vi "Open PolarizationProcessor.vi"(8 "error in (no error)":errorcluster, 11 "PolarizationProcessorSDK reference":refnum<k24>) -> (0 "error out":errorcluster, 2 "PolarizationProcessor reference":refnum<k24>, 3 "PolarizationProcessorSDK reference out":refnum<k24>)   [LabVIEW 2015]
uses:
  C:/code/Host/Installer/Scientific Camera Interfaces/LabVIEW/32_bit/Library_X86/Thorlabs.TSI.PolarizationProcessor.dll
  code/Host/Installer/Scientific Camera Interfaces/LabVIEW/32_bit/Library_X86/Thorlabs.TSI.PolarizationProcessor.dll
  C:/code/Host/Installer/Scientific Camera Interfaces/LabVIEW/32_bit/Library_X86/Thorlabs.TSI.PolarizationInterfaces.dll
  code/Host/Installer/Scientific Camera Interfaces/LabVIEW/32_bit/Library_X86/Thorlabs.TSI.PolarizationInterfaces.dll
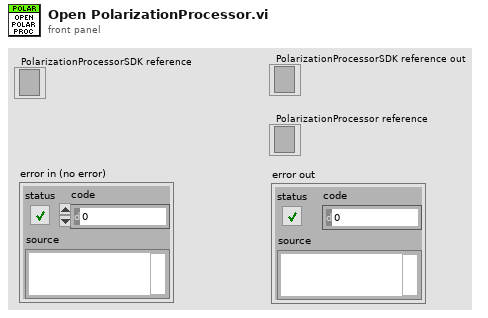
[diagram p1: front panel]
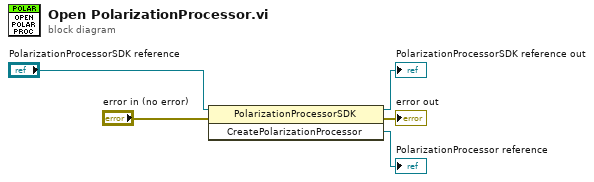
[diagram p0: block diagram]
diagram:
  n1 = invoke class="PolarizationProcessorSDK" method="CreatePolarizationProcessor"(reference="PolarizationProcessorSDK reference", error in="error in (no error)") -> (reference out=→"PolarizationProcessorSDK reference out":refnum<k24>, error out=→"error out":errorcluster, "CreatePolarizationProcessor"=→"PolarizationProcessor reference":refnum<k24>)  [unwired: 1 in]
